vi "DisplayData.vi"(11 "CSV Input":string) -> (3 "Published Data":string[][](array[string]))   [LabVIEW 2015]
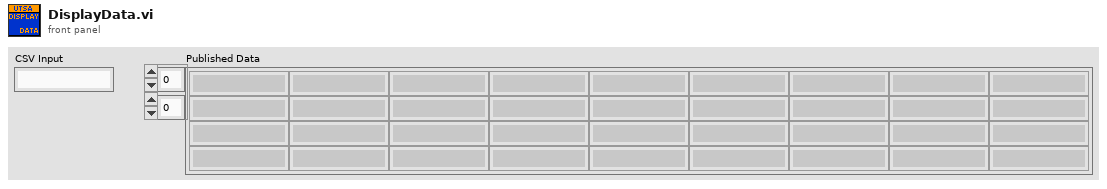
[diagram p1: front panel]
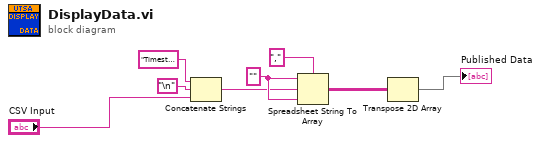
[diagram p0: block diagram]
diagram:
  w6 = "" ("format string")
  n1 = Concatenate Strings("Timestamp,Wind Speed,Wind Direction,Air Pressure,Air Temperature,Internal Temperature,Relative Humidity,Rain Duration, Rain Intensity,Hail Duration, Hail Intensity, Supply Voltage, Irradiance" ("string"), "\n", "CSV Input") -> (w5:string)
  n2 = Spreadsheet String To Array(delimiter (Tab)=",", format string=w6, spreadsheet string=w5, array type (2D Dbl)=w6) -> (array=w7:string[][])
  n3 = Transpose 2D Array(2D array=w7) -> (transposed array=→"Published Data":string[][])
